vi "IMAQdx Snap2.vi"(7 "Timeout (ms)":i32=5000, 8 "error in":errorcluster, 10 "Image In":T2, 11 "Session In":T1) -> (0 "error out":errorcluster, 2 "Image Out":T2, 3 "Session Out":T1)   [LabVIEW 2020, in "NI_Vision_Acquisition_Software.lvlib"]
doc: "Configures, starts, acquires, and unconfigures a snap acquisition. Use a snap for low-speed or single-capture applications where ease of programming is essential. If you call this VI before calling IMAQdx Open Camera.vi, IMAQdx Snap2.vi uses cam0 by default. If the image type does not match the video format of the camera, this VI changes the image type to a suitable format."
uses:
  NI_Vision_Acquisition_Software.lvlib
  IMAQdx.ctl
  IMAQ Image.ctl
  IMAQdx Acquisition Mode.ctl
  IMAQdx Buffer Number Mode.ctl
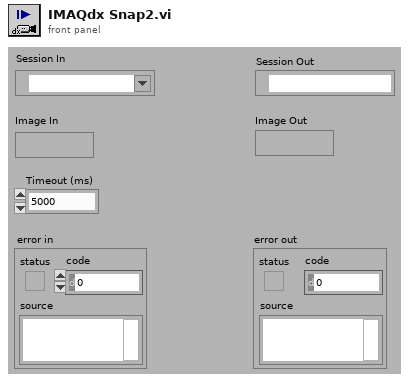
[diagram p1: front panel]
types:
  T1 = typedef "IMAQdx.ctl" = refnum<k21>
  T2 = typedef "IMAQ Image.ctl" = refnum<image>
  T3 = typedef "NI_Vision_Acquisition_Software.lvlib/IMAQdx Buffer Number Mode.ctl" = enum32{"Next", "Last", "Buffer Number", "Every", "Last New"}
  T4 = typedef "NI_Vision_Acquisition_Software.lvlib/IMAQdx Acquisition Mode.ctl" = enum32{"One Shot", "Continuous"}
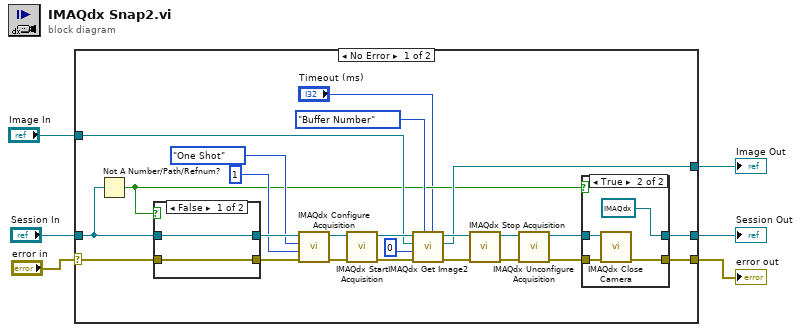
[diagram p0: block diagram]
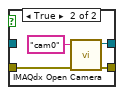
[diagram p3: hidden frame]
diagram:
  n1 = case shown="No Error" "error in" {
    selector: "error in" -> [w7 w43]
    tunnel: "Session In" -> [w29 w44]
    tunnel: "Image In" -> [w21 w45]
    tunnel: [w16 w45] -> w4
    tunnel: [w10 w44] -> w3
    tunnel: [w9 w43] -> w2
    frame No Error {
      n2 = Not A Number/Path/Refnum?(number/path/refnum=w29) -> (NaN/Path/Refnum?=w11:bool)
      n3 = case shown="False" w11 {
        tunnel: [w38 w42] -> w30
        tunnel: w29 -> [w38 _]
        tunnel: [w37 w41] -> w28
        tunnel: w7 -> [w37 w40]
        frame False {
        }
        frame True {
          n4 = call "IMAQdx Open Camera.vi"("error in"=w40, "Session In"="cam0") -> ("error out"=w41:errorcluster, "Session Out"=w42:T1)  [unwired: 8 in]
        }
      }
      n5 = call "IMAQdx Configure Acquisition.vi"("error in"=w28, "Number of Buffers"=u32 1, "Continuous?"=IMAQdx_Acquisition_Mode."One Shot", "Session In"=w30) -> ("error out"=w24:errorcluster, "Session Out"=w25:T1)  [unwired: 6 in]
      n6 = call "IMAQdx Start Acquisition.vi"("error in"=w24, "Session In"=w25) -> ("error out"=w22:errorcluster, "Session Out"=w23:T1)  [unwired: 8 in]
      n7 = call "IMAQdx Get Image2.vi"("Timeout (ms)"="Timeout (ms)", "Buffer Number Mode (Next)"=IMAQdx_Buffer_Number_Mode."Buffer Number" ("Buffer Number Mode"), "error in"=w22, "Buffer Number In"=u32 0, "Image In"=w21, "Session In"=w23) -> ("error out"=w17:errorcluster, "Image Out"=w16:T2, "Session Out"=w18:T1)  [unwired: 2 in, 1 out]
      n8 = call "IMAQdx Stop Acquisition.vi"("error in"=w17, "Session In"=w18) -> ("error out"=w14:errorcluster, "Session Out"=w15:T1)  [unwired: 8 in]
      n9 = call "IMAQdx Unconfigure Acquisition.vi"("error in"=w14, "Session In"=w15) -> ("error out"=w13:errorcluster, "Session Out"=w12:T1)  [unwired: 8 in]
      n10 = case shown="True" w11 {
        tunnel: w13 -> [w31 w36]
        tunnel: w12 -> [w32 w34]
        tunnel: [w32 T1 refnum ("Session Out")] -> w10
        tunnel: [w31 w35] -> w9
        frame False {
        }
        frame True {
          n11 = call "IMAQdx Close Camera.vi"("error in"=w36, "Session In"=w34) -> ("error out"=w35:errorcluster)  [unwired: 9 in]
        }
      }
    }
    frame Error {
    }
  }
  "Image Out" <- w4
  "Session Out" <- w3
  "error out" <- w2
